vi "Write Camera Settings.vi"(8 "error in (no error)":errorcluster, 10 "Camera Settings":variant, 11 "HIJ IMAQdx Display in":refnum<class "HIJ IMAQdx Display.lvclass">) -> (0 "error out":errorcluster, 3 "HIJ IMAQdx Display out":refnum<class "HIJ IMAQdx Display.lvclass">)   [LabVIEW 2014, in "HIJ IMAQdx Display.lvlib" / "HIJ IMAQdx Display.lvclass"]
uses:
  HIJ IMAQdx Display.lvclass
  HIJ IMAQdx Display.lvclass/HIJ IMAQdx Display.ctl
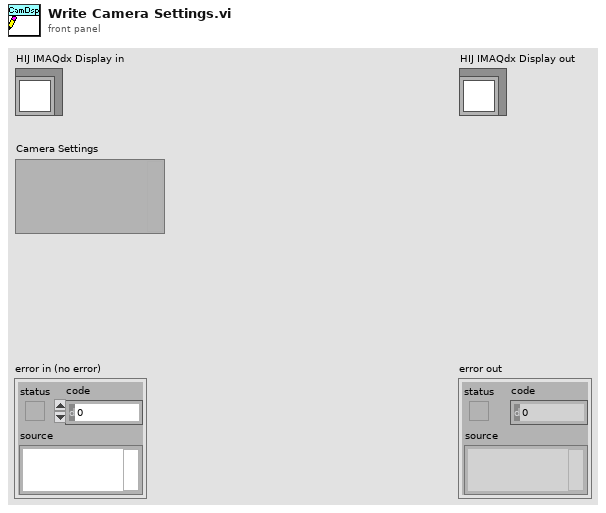
[diagram p1: front panel]
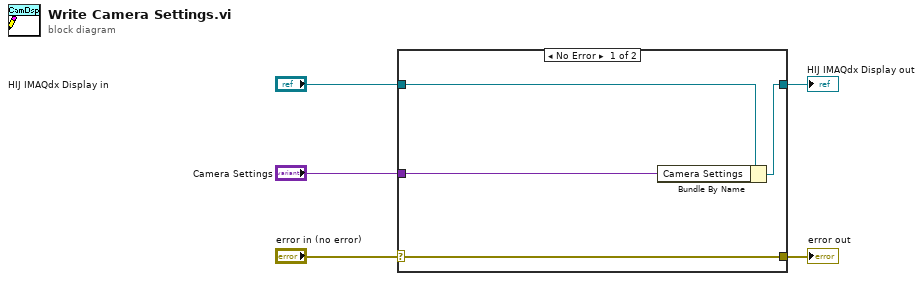
[diagram p0: block diagram]
diagram:
  n1 = case shown="No Error" "error in (no error)" {
    selector: "error in (no error)" -> [w9 w10]
    tunnel: [w9 w10] -> w4
    tunnel: [w7 w11] -> w2
    tunnel: "HIJ IMAQdx Display in" -> [w8 w11]
    tunnel: "Camera Settings" -> [w6 _]
    frame No Error {
      n2 = Bundle By Name(cluster=w8, "Camera Settings"=w6) -> (w7:refnum<class "HIJ IMAQdx Display.lvclass">)
    }
    frame Error {
    }
  }
  "error out" <- w4
  "HIJ IMAQdx Display out" <- w2
